vi "HEWH Calibration Delete Unused String Lines.vi"(11 "Total Array":string[][](array[string])) -> (3 "Output Array":string[][](array[string]))   [LabVIEW 2014]
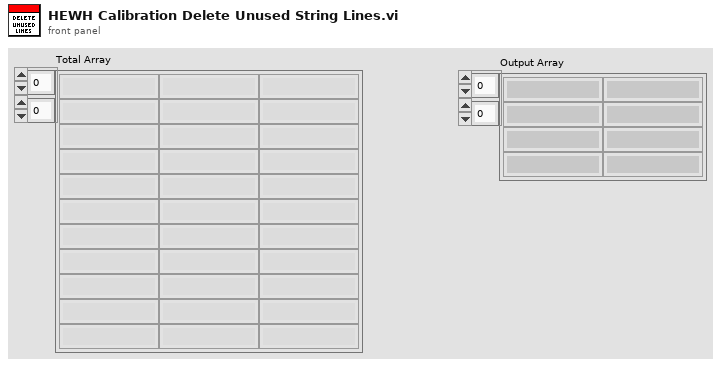
[diagram p1: front panel]
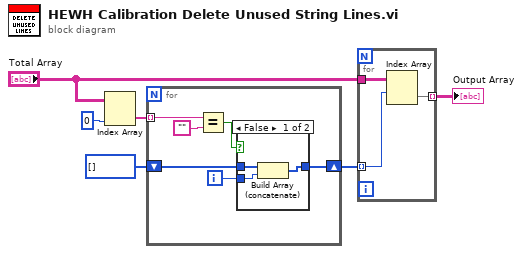
[diagram p0: block diagram]
diagram:
  n1 = Index Array(array="Total Array", index (col)=0 ("disabled index (col)")) -> (element=w5:string[])  [unwired: 1 in]
  n2 = for {
    tunnel: w5 -> [w11] mode=indexing
    shift-right: [w7] -> w2
    shift-left: i32[] [] -> [w8]
    i -> [w9]
    n3 = Equal?(x=w11, y="") -> (x = y?=w10:bool)
    n4 = case shown="False" w10 {
      tunnel: w9 -> [w15 _]
      tunnel: w8 -> [w14 w16]
      tunnel: [w13 w16] -> w7
      frame False {
        n5 = Build Array (concatenate)(w14, w15) -> (w13:i32[])
      }
      frame True {
      }
    }
  }
  n6 = for {
    tunnel: "Total Array" -> [w19]
    tunnel: w2 -> [w18] mode=indexing
    tunnel: [w17] -> w1 mode=indexing
    n7 = Index Array(array=w19, index (row)=w18) -> (element=w17:string[])  [unwired: 1 in]
  }
  "Output Array" <- w1
